vi "Send Thread.vi"(9 "SendQueue":refnum<queue>, 10 "StopNotifier":refnum<notifier>, 11 "Send Data":T1={"Handle"=0, "Frames"=0, "Spare"=0, "Times"=0, "ID+"=FALSE, "Data+"=FALSE, "Type"=enum."CANFD", "Data"=variant}) -> ()   [LabVIEW 2018, in "CAN FD.lvlib"]
uses:
  CAN FD.lvlib
  Typedef/Send Data.ctl
  data_type/ZCAN_Transmit_Data.ctl
  data_type/ZCAN_TransmitFD_Data.ctl
  SubVI/zlgcan.lvlib
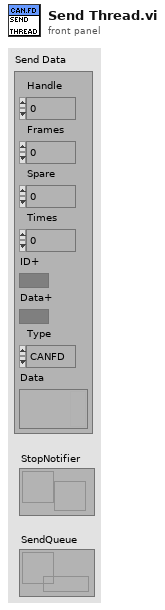
[diagram p1: front panel]
types:
  T1 = typedef "CAN FD.lvlib/Send Data.ctl" = cluster{"Handle":u64, "Frames":u32, "Spare":u32, "Times":i32, "ID+":bool, "Data+":bool, "Type":enum16{"CAN", "CANFD"}, "Data":variant}
  T2 = typedef "ZCAN_Transmit_Data.ctl" = cluster{"帧类型":u32, "帧格式":u32, "ID":u32, "数据长度":u8, "DATA":cluster{"CAN数据[0]":u8, "CAN数据[1]":u8, "CAN数据[2]":u8, "CAN数据[3]":u8, "CAN数据[4]":u8, "CAN数据[5]":u8, "CAN数据[6]":u8, "CAN数据[7]":u8}, "发送方式":u32}
  T3 = typedef "ZCAN_TransmitFD_Data.ctl" = cluster{"帧类型":u32, "帧格式":u32, "ID":u32, "数据长度":u8, "CANFD加速？":u8, "DATA":cluster{"CAN数据[0]":u8, "CAN数据[1]":u8, "CAN数据[2]":u8, "CAN数据[3]":u8, "CAN数据[4]":u8, "CAN数据[5]":u8, "CAN数据[6]":u8, "CAN数据[7]":u8, "CAN数据[8]":u8, "CAN数据[9]":u8, "CAN数据[10]":u8, "CAN数据[11] ":u8, "CAN数据[12] ":u8, "CAN数据[13] ":u8, "CAN数据[14] ":u8, "CAN数据[15] ":u8, "CAN数据[16]":u8, "CAN数据[17]":u8, "CAN数据[18]":u8, "CAN数据[19]":u8, "CAN数据[20]":u8, "CAN数据[21]":u8, "CAN数据[22]":u8, "CAN数据[23]":u8, "CAN数据[24] ":u8, "CAN数据[25]":u8, "CAN数据[26]":u8, "CAN数据[27]":u8, "CAN数据[28]":u8, "CAN数据[29]":u8, "CAN数据[30]":u8, "CAN数据[31]":u8, "CAN数据[32]":u8, "CAN数据[33]":u8, "CAN数据[34]":u8, "CAN数据[35]":u8, "CAN数据[36]":u8, "CAN数据[37]":u8, "CAN数据[38]":u8, "CAN数据[39]":u8, "CAN数据[40]":u8, "CAN数据[41]":u8, "CAN数据[42]":u8, "CAN数据[43]":u8, "CAN数据[44]":u8, "CAN数据[45]":u8, "CAN数据[46]":u8, "CAN数据[47]":u8, "CAN数据[48]":u8, "CAN数据[49]":u8, "CAN数据[50]":u8, "CAN数据[51]":u8, "CAN数据[52]":u8, "CAN数据[53]":u8, "CAN数据[54]":u8, "CAN数据[55]":u8, "CAN数据[56]":u8, "CAN数据[57]":u8, "CAN数据[58]":u8, "CAN数据[59]":u8, "CAN数据[60]":u8, "CAN数据[61]":u8, "CAN数据[62]":u8, "CAN数据[63]":u8}, "发送方式":u32}
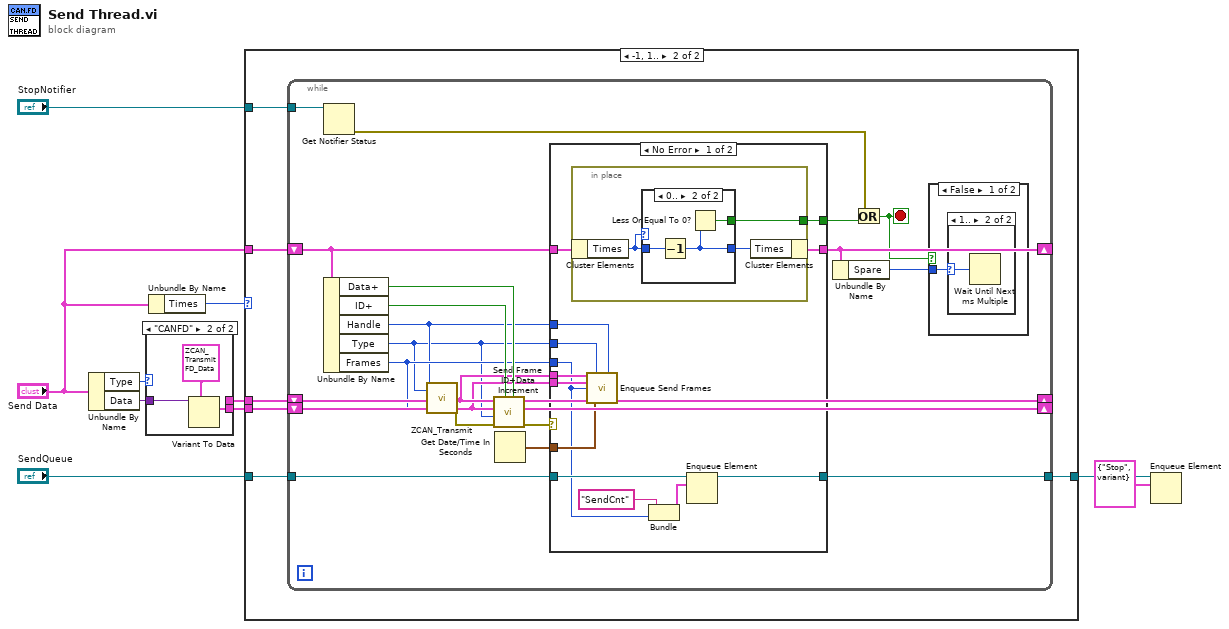
[diagram p0: block diagram]
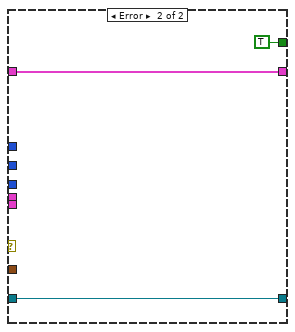
[diagram p6: hidden frame]
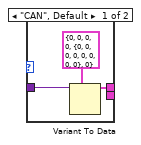
[diagram p7: hidden frame]
diagram:
  n1 = Unbundle By Name("Send Data") -> ("Type"=w6:enum16{"CAN", "CANFD"}, "Data"=w9:variant)
  n2 = case shown="\"CANFD\"" w6 {
    tunnel: w9 -> [w13 w16]
    tunnel: [w11 _] -> w8
    tunnel: [_ w14] -> w7
    frame "CAN", Default {
      n3 = Variant To Data(type=T2 {"帧类型"=0, "帧格式"=0, "ID"=0, "数据长度"=0, "DATA"={"CAN数据[0]"=0, "CAN数据[1]"=0, "CAN数据[2]"=0, "CAN数据[3]"=0, "CAN数据[4]"=0, "CAN数据[5]"=0, "CAN数据[6]"=0, "CAN数据[7]"=0}, "发送方式"=0} ("ZCAN_Transmit_Data"), Variant=w13) -> (data=w11:T2)  [unwired: 1 in, 1 out]
    }
    frame "CANFD" {
      n4 = Variant To Data(type=T3 {"帧类型"=0, "帧格式"=0, "ID"=0, "数据长度"=0, "CANFD加速？"=0, "DATA"={"CAN数据[0]"=0, "CAN数据[1]"=0, "CAN数据[2]"=0, "CAN数据[3]"=0, "CAN数据[4]"=0, "CAN数据[5]"=0, "CAN数据[6]"=0, "CAN数据[7]"=0, "CAN数据[8]"=0, "CAN数据[9]"=0, "CAN数据[10]"=0, "CAN数据[11] "=0, "CAN数据[12] "=0, "CAN数据[13] "=0, "CAN数据[14] "=0, "CAN数据[15] "=0, "CAN数据[16]"=0, "CAN数据[17]"=0, "CAN数据[18]"=0, "CAN数据[19]"=0, "CAN数据[20]"=0, "CAN数据[21]"=0, "CAN数据[22]"=0, "CAN数据[23]"=0, "CAN数据[24] "=0, "CAN数据[25]"=0, "CAN数据[26]"=0, "CAN数据[27]"=0, "CAN数据[28]"=0, "CAN数据[29]"=0, "CAN数据[30]"=0, "CAN数据[31]"=0, "CAN数据[32]"=0, "CAN数据[33]"=0, "CAN数据[34]"=0, "CAN数据[35]"=0, "CAN数据[36]"=0, "CAN数据[37]"=0, "CAN数据[38]"=0, "CAN数据[39]"=0, "CAN数据[40]"=0, "CAN数据[41]"=0, "CAN数据[42]"=0, "CAN数据[43]"=0, "CAN数据[44]"=0, "CAN数据[45]"=0, "CAN数据[46]"=0, "CAN数据[47]"=0, "CAN数据[48]"=0, "CAN数据[49]"=0, "CAN数据[50]"=0, "CAN数据[51]"=0, "CAN数据[52]"=0, "CAN数据[53]"=0, "CAN数据[54]"=0, "CAN数据[55]"=0, "CAN数据[56]"=0, "CAN数据[57]"=0, "CAN数据[58]"=0, "CAN数据[59]"=0, "CAN数据[60]"=0, "CAN数据[61]"=0, "CAN数据[62]"=0, "CAN数据[63]"=0}, "发送方式"=0} ("ZCAN_TransmitFD_Data"), Variant=w16) -> (data=w14:T3)  [unwired: 1 in, 1 out]
    }
  }
  n5 = Unbundle By Name("Send Data") -> ("Times"=w1:i32)
  n6 = case shown="-1, 1.." w1 {
    tunnel: "StopNotifier" -> [_ w23]
    tunnel: w8 -> [_ w22]
    tunnel: w7 -> [_ w21]
    tunnel: "SendQueue" -> [w17 w20]
    tunnel: [w17 w19] -> w4
    tunnel: "Send Data" -> [_ w18]
    frame 0, Default {
    }
    frame -1, 1.. {
      n7 = while {
        tunnel: w23 -> [w44]
        shift-right: [w41] -> _
        shift-left: w22 -> [w36]
        shift-right: [w40] -> _
        shift-left: w21 -> [w35]
        shift-right: [w26] -> _
        shift-left: w18 -> [w37]
        tunnel: w20 -> [w30]
        tunnel: [w27] -> w19
        stop <- w25 stop-if-true
        n8 = Get Notifier Status(notifier=w44) -> (error out=w28:errorcluster)  [unwired: 1 in, 4 out]
        n9 = Unbundle By Name(w37) -> ("Data+"=w42:bool, "ID+"=w43:bool, "Handle"=w33:u64, "Type"=w31:enum16{"CAN", "CANFD"}, "Frames"=w34:u32)
        n10 = call "ZCAN_Transmit.vi"("can_index_handle"=w33, "协议"=w31, "ZCAN_Transmit_Data"=w36, "每次发送帧数（默认1）"=w34, "ZCAN_TransmitFD_Data"=w35) -> ("error out"=w39:errorcluster)  [unwired: 14 in]
        n11 = call "Send Frame ID+Data Increment.vi"("Data+"=w42, "ID+"=w43, "error in (no error)"=w39, "Protocol"=w31, "ZCAN_TransmitFD_Data"=w35, "ZCAN_Transmit_Data"=w36) -> ("error out"=w38:errorcluster, "ZCAN_TransmitFD_Data out"=w40:T3, "ZCAN_Transmit_Data out"=w41:T2)  [unwired: 3 in]
        n12 = Get Date/Time In Seconds() -> (seconds since 1Jan1904=w32:timestamp)
        n13 = case shown="No Error" w38 {
          tunnel: w37 -> [w59 w69]
          tunnel: [w58 w69] -> w26
          tunnel: [w57 TRUE] -> w29
          tunnel: w36 -> [w56 _]
          tunnel: w35 -> [w55 _]
          tunnel: w34 -> [w50 _]
          tunnel: w33 -> [w52 _]
          tunnel: w32 -> [w54 _]
          tunnel: w31 -> [w53 _]
          tunnel: w30 -> [w51 w67]
          tunnel: [w47 w67] -> w27
          frame No Error {
            n14 = in-place {
              in-place-border: [w61] -> w57
              n15 = in-place-cluster #1(w59) -> ("Times"=w60:i32)
              n16 = case shown="0.." w60 {
                tunnel: w60 -> [w63 w66]
                tunnel: [w63 w65] -> w62
                tunnel: [_ w64] -> w61
                frame -1, Default {
                }
                frame 0.. {
                  n17 = Decrement(x=w66) -> (x-1=w65:i32)
                  n18 = Less Or Equal To 0?(x=w65) -> (x <= 0?=w64:bool)
                }
              }
              n19 = in-place-cluster #1("Times"=w62) -> (w58:T1)
            }
            n20 = call "Enqueue Send Frames.vi"("ZCAN_Transmit_Data"=w56, "Protocol"=w53, "ChannelHandle"=w52, "ZCAN_TransmitFD_Data"=w55, "Frames"=w50, "Timestamp"=w54) -> ()  [unwired: 10 in]
            n21 = Bundle("SendCnt", "Frames"=w50) -> (w48:cluster{string, "Frames":u32})  [unwired: 1 in]
            n22 = Enqueue Element(queue=w51, element=w48) -> (queue out=w47:refnum<queue>)  [unwired: 2 in, 2 out]
          }
          frame Error {
          }
        }
        n23 = Unbundle By Name(w26) -> ("Spare"=w24:u32)
        n24 = Or(x=w28, y=w29) -> (x .or. y?=w25:bool)
        n25 = case shown="False" w25 {
          tunnel: w24 -> [w45 _]
          frame False {
            n26 = case shown="1.." w45 {
              selector: w45 -> [_ w46]
              frame 0, Default {
              }
              frame 1.. {
                n27 = Wait Until Next ms Multiple(millisecond multiple=w46) -> ()  [unwired: 1 out]
              }
            }
          }
          frame True {
          }
        }
      }
    }
  }
  n28 = Enqueue Element(queue=w4, element=cluster{"ID":string, "Data":variant} {"ID"="Stop", "Data"=variant} ("元素")) -> ()  [unwired: 2 in, 3 out]
